vi "load varpolydelay.vi"(8 "error in (no error)":errorcluster, 10 "tableno":u16, 11 "stbfilename":string) -> (0 "error out":errorcluster, 3 "function return":i16)   [LabVIEW 2015, in "SCANalone4x64.lvlib"]
doc: "__declspec(dllimport) short __stdcall load_varpolydelay(const char* stbfilename, unsigned short tableno);"
uses:
  <userlib>/SCANalone4x64/SCANalone4x64.lvlib
  <userlib>/SCANalone4x64/SCANalone4x64.dll
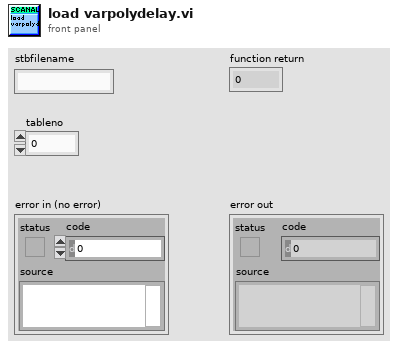
[diagram p1: front panel]
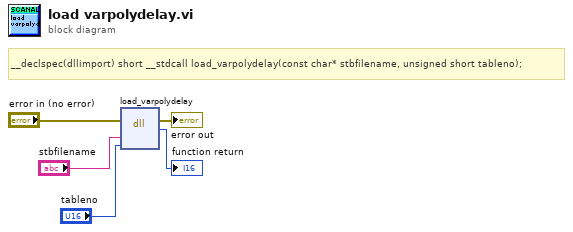
[diagram p0: block diagram]
diagram:
  # "__declspec(dllimport) short __stdcall load_varpolydelay(const char* stbfilename, unsigned short tableno);"
  n1 = dll-call lib="C:/Program Files/National Instruments/LabVIEW 2015/user.lib/SCANalone4x64/SCANalone4x64.*" fn="load_varpolydelay"(error in="error in (no error)", "stbfilename"="stbfilename", "tableno"="tableno") -> (error out=→"error out":errorcluster, →"function return":i16)  [unwired: 4 in, 1 out]
